vi "Subscribe Observer.vi"(8 "error in (no error)":errorcluster, 10 "Device Connector MSG In":refnum<class "Device Connector MSG.lvclass">, 11 "Device Connector in":refnum<class "Device Connector.lvclass">) -> (0 "error out":errorcluster, 3 "Device Connector out":refnum<class "Device Connector.lvclass">)   [LabVIEW 2024, in "Device Connector.lvclass"]
uses:
  Device Connector.lvclass
  Device Connector MSG/Device Connector MSG.lvclass
  C:/Users/iio/Desktop/Bussiness/Tricorn Re/Madelbrot 4.0/General Library/Ancestor Class/Message/Message.lvclass
  Device Connector.lvclass/Device Connector.ctl
  Ancestor Class/Message/Message.lvclass/Message.ctl
  Ancestor Class/Message/Public Data/Read Subscriber.vi
  Ancestor Class/Actor Assistant/Subscriber/Subscriber.lvclass
  Ancestor Class/Actor Assistant/Observer/Observer.lvclass
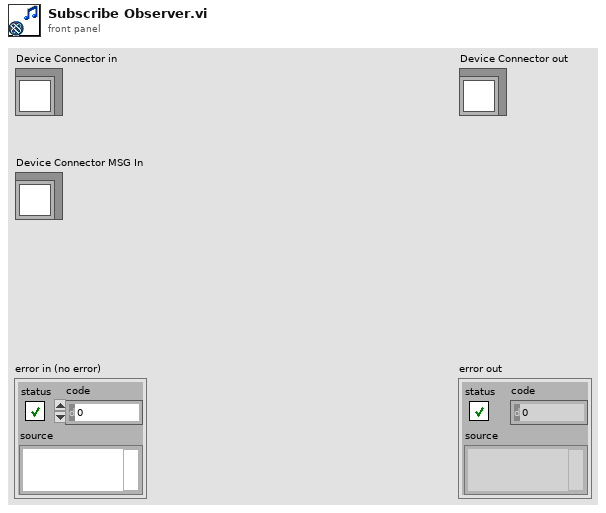
[diagram p1: front panel]
types:
  T1 = typedef "Observer Queue.ctl" = refnum<queue>
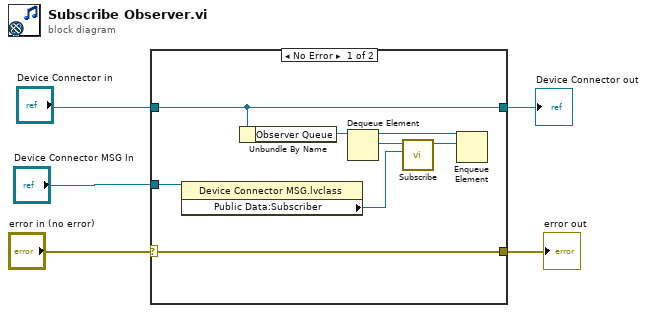
[diagram p0: block diagram]
diagram:
  n1 = case shown="No Error" "error in (no error)" {
    selector: "error in (no error)" -> [w13 w15]
    tunnel: [w13 w15] -> w4
    tunnel: [w6 w14] -> w2
    tunnel: "Device Connector in" -> [w6 w14]
    tunnel: "Device Connector MSG In" -> [w12 _]
    frame No Error {
      n2 = property class="Device Connector MSG.lvclass"(reference=w12) -> ("Public Data:Subscriber"=w11:refnum<class "Subscriber.lvclass">)  [unwired: 1 in, 2 out]
      n3 = Unbundle By Name(w6) -> ("Observer Queue"=w10:T1)
      n4 = Dequeue Element(queue=w10) -> (queue out=w7:T1, element=w9:refnum<class "Observer.lvclass">)  [unwired: 2 in, 2 out]
      n5 = call-dynamic "Subscribe.vi"("Subscriber In"=w11, "Observer in"=w9) -> ("Observer out"=w8:refnum<class "Observer.lvclass">)  [unwired: 8 in, 1 out]
      n6 = Enqueue Element(queue=w7, element=w8) -> ()  [unwired: 2 in, 3 out]
    }
    frame Error {
    }
  }
  "error out" <- w4
  "Device Connector out" <- w2
